vi "Clear HW Torque Trim Sensors 5.vi"(6 "error in":errorcluster, 8 "MaxRead":i32, 9 "Channel in":u16) -> (0 "error out":errorcluster, 1 "Messages":T1(array[cluster]) {"DATA[1]" format="%.0x"; "DATA[3]" format="%.0x"; "DATA[4]" format="%.0x"}, 2 "Pass":bool, 3 "Channel out":u16)   [LabVIEW 2023]
uses:
  4f930f32-d09a-43ef-bca1-8b214b378bd5.vi
  ca49bb01-4f9d-4fc6-af7c-560520f89dfa.vi
  Communication/PCAN2023/PCAN API.lvlib
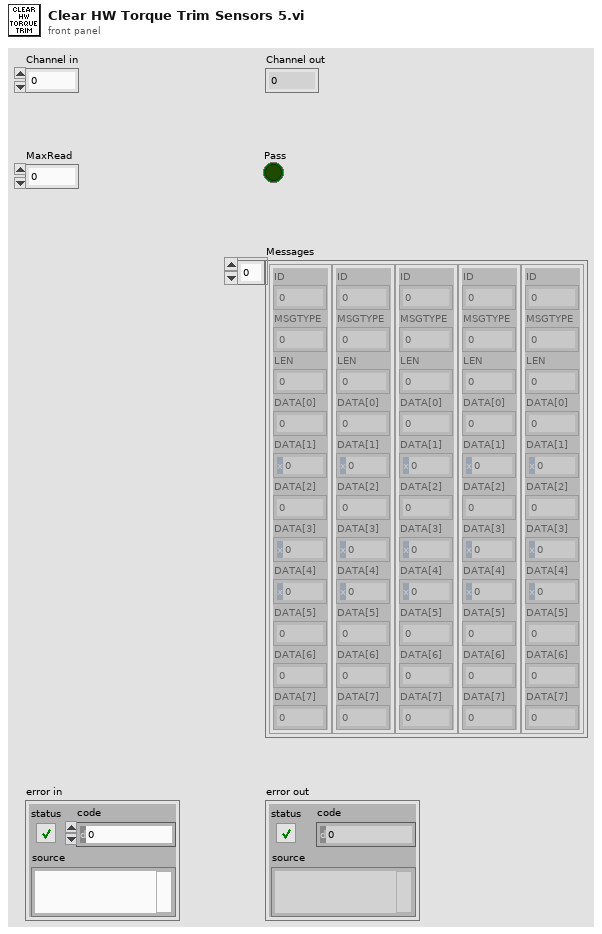
[diagram p1: front panel]
types:
  T1 = cluster{"ID":u32, "MSGTYPE":u8, "LEN":u8, "DATA[0]":u8, "DATA[1]":u8, "DATA[2]":u8, "DATA[3]":u8, "DATA[4]":u8, "DATA[5]":u8, "DATA[6]":u8, "DATA[7]":u8}[]
  T2 = cluster{"ID":u32, "MSGTYPE":u8, "LEN":u8, "DATA[0]":u8, "DATA[1]":u8, "DATA[2]":u8, "DATA[3]":u8, "DATA[4]":u8, "DATA[5]":u8, "DATA[6]":u8, "DATA[7]":u8}
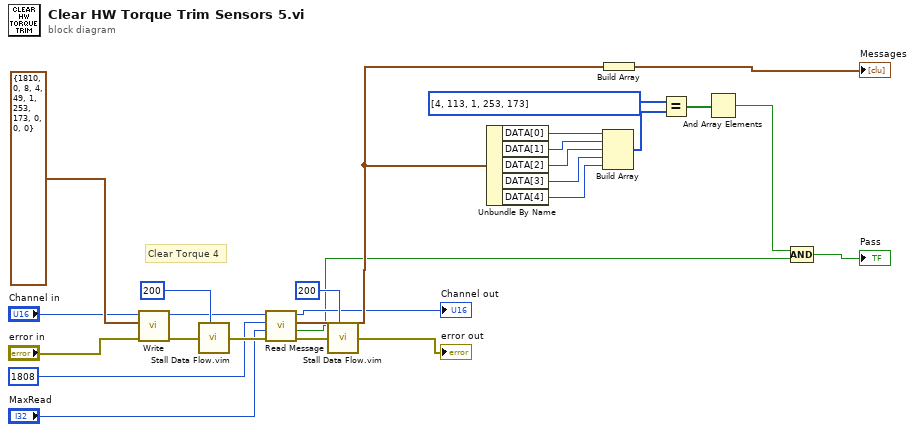
[diagram p0: block diagram]
diagram:
  # "Clear Torque 4"
  n1 = call "Write.vi"("error in"="error in", "MessageBuffer"=T2 {"ID"=1810, "MSGTYPE"=0, "LEN"=8, "DATA[0]"=4, "DATA[1]"=49, "DATA[2]"=1, "DATA[3]"=253, "DATA[4]"=173, "DATA[5]"=0, "DATA[6]"=0, "DATA[7]"=0}, "Channel"="Channel in") -> ("error out"=w22:errorcluster, "Channel out"=w10:u16)  [unwired: 5 in, 2 out]
  n2 = call "Stall Data Flow.vim"("value in"=w22, "milliseconds to wait"=u32 200) -> ("value out"=w9:errorcluster)  [unwired: 1 out]
  n3 = call "Read Message.vi"("error in"=w9, "MaxRead"="MaxRead", "ID"=u32 1808, "Channel in"=w10) -> ("error out"=w8:errorcluster, "Passed"=w1:bool, "Last Message"=w7:T2, "Channel out"=→"Channel out":u16)  [unwired: 3 in, 1 out]
  n4 = call "Stall Data Flow.vim"("value in"=w8, "milliseconds to wait"=u32 200) -> ("value out"=→"error out":errorcluster)  [unwired: 1 out]
  n5 = Unbundle By Name(w7) -> ("DATA[0]"=w20:u8, "DATA[1]"=w19:u8, "DATA[2]"=w18:u8, "DATA[3]"=w15:u8, "DATA[4]"=w14:u8)
  n6 = Build Array(w20, w19, w18, w15, w14) -> (w12:u8[])
  n7 = Build Array(w7) -> (→"Messages":T1)
  n8 = Equal?(x=u8[] [4, 113, 1, 253, 173] ("y"), y=w12) -> (x = y?=w11:bool[])
  n9 = And Array Elements(Boolean array=w11) -> (logical AND=w4:bool)
  n10 = Compound Arithmetic op=AND(w4, w1) -> (→"Pass":bool)
